vi "FPGA_DMAConfigureHostBuffer.vi"(8 "error in (no error)":errorcluster, 10 "Depth":u32=10000, 11 "DMADevRef In":T1) -> (0 "error out":errorcluster, 3 "DMADevRef Out":T1)   [LabVIEW 2017]
uses:
  <vilib>/Rock Robotics/SystemInterfaces/DMA/FPGA_DMADevRef.ctl
  <vilib>/Rock Robotics/SystemInterfaces/System/FPGA_SystemFPGA Ref Global.vi
  <vilib>/rvi/interface/common/niFpgaWaitOnOcc.vi
  <vilib>/Utility/error.llb/Error Cluster From Error Code.vi
  <vilib>/rvi/interface/nirviMethod/nirviMethod.xnode
  <vilib>/Rock Robotics/SystemInterfaces/System/FPGA_SystemFRC FPGA Ref.ctl
  <vilib>/FPGAPlugInAG/Dynamic/niLvFpga_ConfigureFifo_Dynamic.vi
  <vilib>/rvi/errors/niLvFpgaMergeErrorWithErrorCode.vi
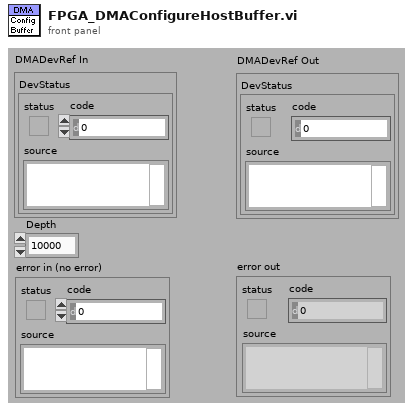
[diagram p1: front panel]
types:
  T1 = typedef "FPGA_DMADevRef.ctl" = cluster{"DevStatus":errorcluster}
  T2 = typedef "FPGA_SystemFRC FPGA Ref.ctl" = refnum<k20>
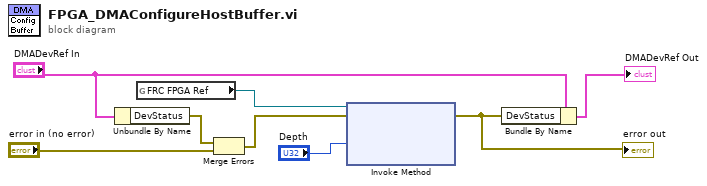
[diagram p0: block diagram]
diagram:
  n1 = Unbundle By Name("DMADevRef In") -> ("DevStatus"=w4:errorcluster)
  n2 = global read "FPGA_SystemFPGA Ref Global.vi" "FRC FPGA Ref"() -> (w1:T2)
  n3 = Merge Errors(w4, "error in (no error)") -> (w2:errorcluster)
  n4 = xnode "Invoke Method"("FPGA VI Reference In"=w1, "error in"=w2, "Requested Depth"="Depth") -> ("error out"=w6:errorcluster)  [unwired: 2 out]
  "error out" <- w6
  n5 = Bundle By Name(cluster="DMADevRef In", "DevStatus"=w6) -> (→"DMADevRef Out":T1)
